vi "Edit Config.vi"(8 "error in (no error)":errorcluster, 11 "NI Analog in":refnum<class "All Channels Out.lvclass">) -> (0 "error out":errorcluster, 3 "NI Analog out":refnum<class "All Channels Out.lvclass">)   [LabVIEW 2024, in "All Channels Out.lvclass"]
doc: "NI Analog Out.lvclass:Edit Config.vi\n\nThis VI is used to edit the NI Analog Out configuration parameters.\n\nInstrument Communication Module Version 1.0\nOctober, 2020 Original Code Consulting Davita Bird\n www.originalcode.com"
uses:
  All Channels Out.lvclass
  All Channels Type Def.ctl
  ICM Class Editor State.ctl
  ICM Editor Command.ctl
  All Channels Out.lvclass/All Channels Out.ctl
panel:
  in  "All Channels Config":T1
  in  "Flash Save":bool
  in  "Save":bool
  in  "Revert":bool
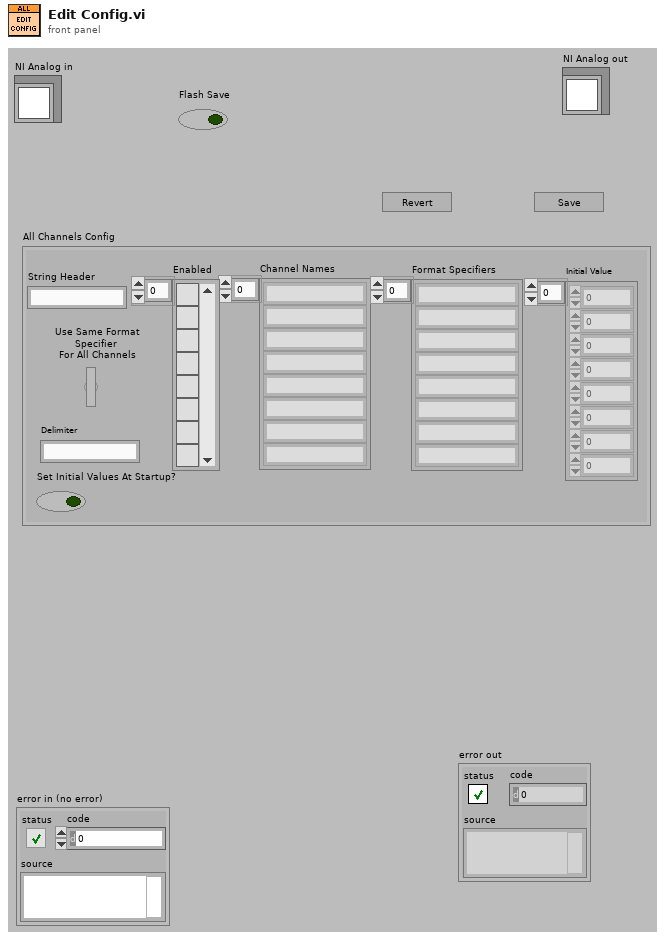
[diagram p1: front panel]
types:
  T1 = typedef "All Channels Type Def.ctl" = cluster{"Channel Names":string[], "Enabled":bool[], "Format Specifiers":string[], "String Header":string, "Use Same Format\nSpecifier \nFor All Channels":bool, "Delimiter":string, "Initial Value":dbl[], "Set Initial Values At Startup?":bool}
  T2 = typedef "ICM Editor Command.ctl" = enum16{"No-op", "Exit"}
  T3 = typedef "ICM Class Editor State.ctl" = enum16{"Init", "Wait", "Write", "Read", "Display", "Set Flashing", "Error", "Stop"}
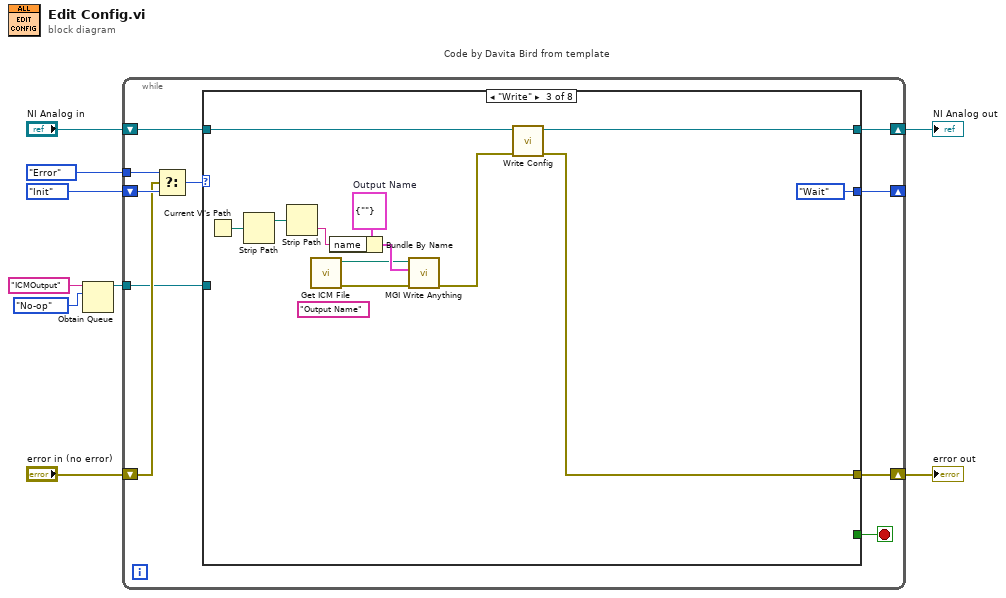
[diagram p0: block diagram]
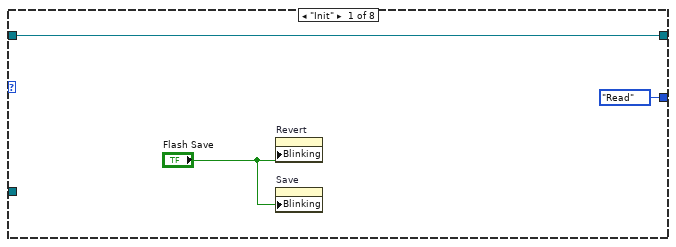
[diagram p2: hidden frame]
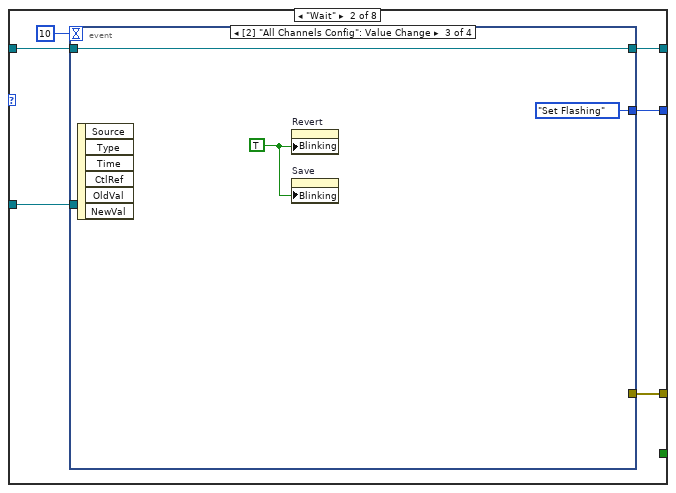
[diagram p3: hidden frame]
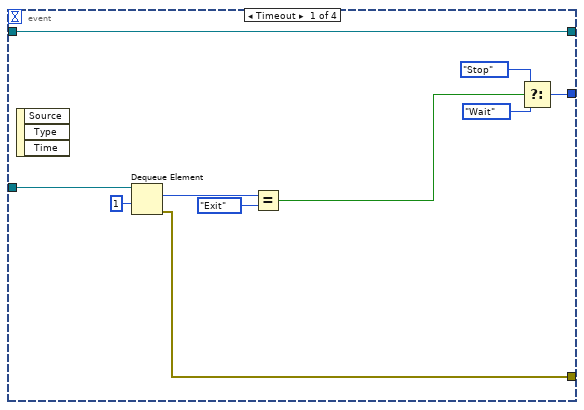
[diagram p4: hidden frame]
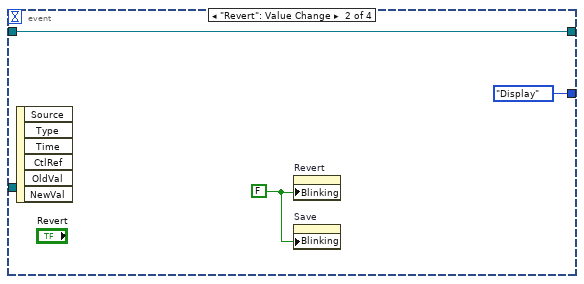
[diagram p5: hidden frame]
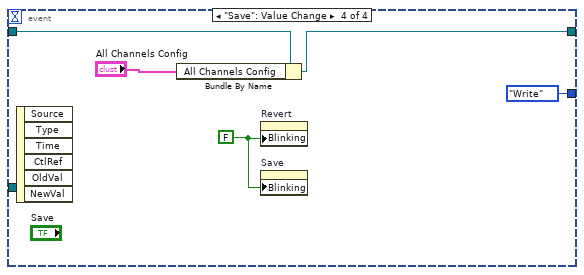
[diagram p6: hidden frame]
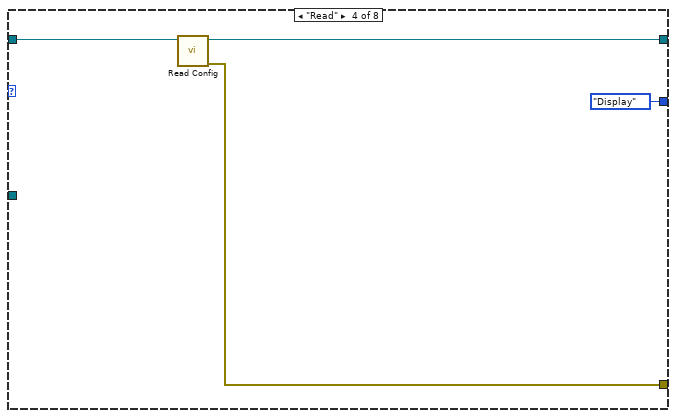
[diagram p7: hidden frame]
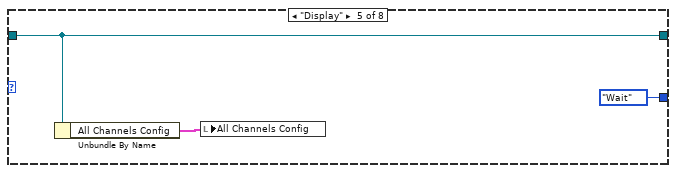
[diagram p8: hidden frame]
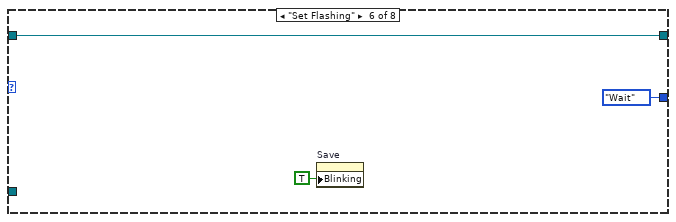
[diagram p9: hidden frame]
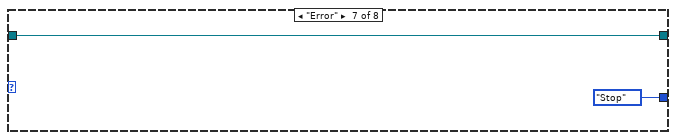
[diagram p10: hidden frame]
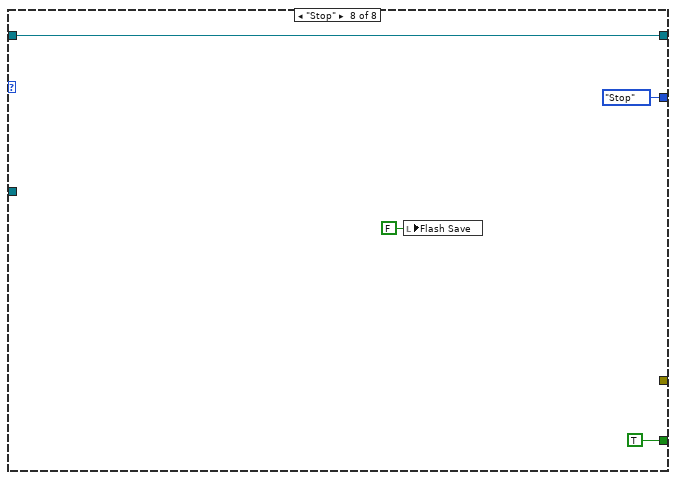
[diagram p11: hidden frame]
diagram:
  n1 = Obtain Queue(name (unnamed)="ICMOutput", element data type=ICM_Editor_Command."No-op" ("Editor Command")) -> (queue out=w1:refnum<queue>)  [unwired: 3 in, 2 out]
  n2 = while "Code by Davita Bird from template" {
    shift-right: [w19] -> w8
    shift-left: "NI Analog in" -> [w18]
    shift-right: [w12] -> _
    shift-left: ICM_Class_Editor_State."Init" ("Config State") -> [w16]
    shift-right: [w11] -> w6
    shift-left: "error in (no error)" -> [w14]
    tunnel: ICM_Class_Editor_State."Error" ("Config State") -> [w13]
    tunnel: w1 -> [w10]
    stop <- w17 stop-if-true
    n3 = Select(t=w13, s=w14, f=w16) -> (s? t:f=w15:T3)
    n4 = case shown="\"Write\"" w15 {
      tunnel: [w21 w26 w59 w63 w68 w71 w73 w77] -> w19
      tunnel: w18 -> [w21 w25 w60 w65 w68 w71 w73 w77]
      tunnel: [_ _ _ _ _ _ _ TRUE] -> w17
      tunnel: [ICM_Class_Editor_State."Read" ("Config State") w27 ICM_Class_Editor_State."Wait" ("Config State") ICM_Class_Editor_State."Display" ("Config State") ICM_Class_Editor_State."Wait" ("Config State") ICM_Class_Editor_State."Wait" ("Config State") ICM_Class_Editor_State."Stop" ("Config State") ICM_Class_Editor_State."Stop" ("Config State")] -> w12
      tunnel: [_ w23 w58 w64 _ _ _ _] -> w11
      tunnel: w10 -> [_ w24 _ _ _ _ _ _]
      frame "Init" {
        n5 = property on="Revert" class="Bool"("Blinking"="Flash Save") -> ()  [unwired: 2 in, 2 out]
        n6 = property on="Save" class="Bool"("Blinking"="Flash Save") -> ()  [unwired: 2 in, 2 out]
      }
      frame "Wait" {
        n7 = event shown="[2] \"All Channels Config\": Value Change" {
          selector: _ -> [_ _ _ _]
          dyn-events: _ -> [_ _ _ _]
          timeout: 10 -> [_ _ _ _]
          tunnel: [w35 ICM_Class_Editor_State."Display" ("Config State") ICM_Class_Editor_State."Set Flashing" ("Config State") ICM_Class_Editor_State."Write" ("Config State")] -> w27
          tunnel: [w38 w40 w44 w47] -> w26
          tunnel: w25 -> [w38 w40 w44 w48]
          tunnel: w24 -> [w37 _ _ _]
          tunnel: [w29 _ _ _] -> w23
          event Timeout {
            n8 = event-data() -> ()  [unwired: 1 in, 3 out]
            n9 = Dequeue Element(queue=w37, timeout in ms (-1)=1) -> (element=w34:T2, error out=w29:errorcluster)  [unwired: 1 in, 2 out]
            n10 = Equal?(x=w34, y=ICM_Editor_Command."Exit") -> (x = y?=w32:bool)
            n11 = Select(t=ICM_Class_Editor_State."Stop" ("Config State"), s=w32, f=ICM_Class_Editor_State."Wait" ("Config State")) -> (s? t:f=w35:T3)
          }
          event "Revert": Value Change {
            w39 = FALSE ("Blinking")
            n12 = event-data() -> ()  [unwired: 1 in, 6 out]
            n13 = property on="Revert" class="Bool"("Blinking"=w39) -> ()  [unwired: 2 in, 2 out]
            n14 = property on="Save" class="Bool"("Blinking"=w39) -> ()  [unwired: 2 in, 2 out]
          }
          event Value Change {
            w42 = TRUE ("Blinking")
            n15 = event-data() -> ()  [unwired: 1 in, 6 out]
            n16 = property on="Revert" class="Bool"("Blinking"=w42) -> ()  [unwired: 2 in, 2 out]
            n17 = property on="Save" class="Bool"("Blinking"=w42) -> ()  [unwired: 2 in, 2 out]
          }
          event "Save": Value Change {
            w46 = FALSE ("Blinking")
            n18 = event-data() -> ()  [unwired: 1 in, 6 out]
            n19 = Bundle By Name(cluster=w48, "All Channels Config"="All Channels Config") -> (w47:refnum<class "All Channels Out.lvclass">)
            n20 = property on="Revert" class="Bool"("Blinking"=w46) -> ()  [unwired: 2 in, 2 out]
            n21 = property on="Save" class="Bool"("Blinking"=w46) -> ()  [unwired: 2 in, 2 out]
          }
        }
      }
      frame "Write" {
        w54 = cluster{"name":string} {"name"=""}  # Output Name
        (unwired) "Output Name" ("Section Name (Name of \"Anything\")")
        n22 = Current VI's Path() -> (path=w57:path)
        n23 = Strip Path(path=w57) -> (stripped path=w56:path)  [unwired: 1 out]
        n24 = Strip Path(path=w56) -> (name=w53:string)  [unwired: 1 out]
        n25 = call "Get ICM File.vi"() -> ("error out"=w55:errorcluster, "ICM File"=w50:path)  [unwired: 10 in]
        n26 = Bundle By Name(cluster=w54, "name"=w53) -> (w52:cluster{"name":string})
        n27 = call "MGI Write Anything.vi"("Error In"=w55, "Anything"=w52, "Path (dialog)"=w50) -> ("Error Out"=w51:errorcluster)  [unwired: 6 in, 2 out]
        n28 = call-dynamic "Write Config.vi"("error in (no error)"=w51, "All Channels in"=w60) -> ("error out"=w58:errorcluster, "All Channels out"=w59:refnum<class "All Channels Out.lvclass">)  [unwired: 8 in]
      }
      frame "Read" {
        n29 = call-dynamic "Read Config.vi"("All Channels in"=w65) -> ("error out"=w64:errorcluster, "All Channels out"=w63:refnum<class "All Channels Out.lvclass">)  [unwired: 9 in]
      }
      frame "Display" {
        n30 = Unbundle By Name(w68) -> ("All Channels Config"=w67:T1)
        n31 = local write "All Channels Config"(w67) -> ()
      }
      frame "Set Flashing" {
        n32 = property on="Save" class="Bool"("Blinking"=TRUE) -> ()  [unwired: 2 in, 2 out]
      }
      frame "Error" {
      }
      frame "Stop" {
        n33 = local write "Flash Save"(FALSE ("Flash Save")) -> ()
      }
    }
  }
  "error out" <- w6
  "NI Analog out" <- w8
